vi "Roller Speeds.vi"(0 "Top In":dbl, 1 "Distance":dbl, 2 "Time Elapsed":bool, 3 "Selector":bool caption="Reset", 4 "Trigger":bool, 5 "Bottom In":dbl) -> (14 "Top Out":dbl, 19 "Bottom Out":dbl)   [LabVIEW 2012]
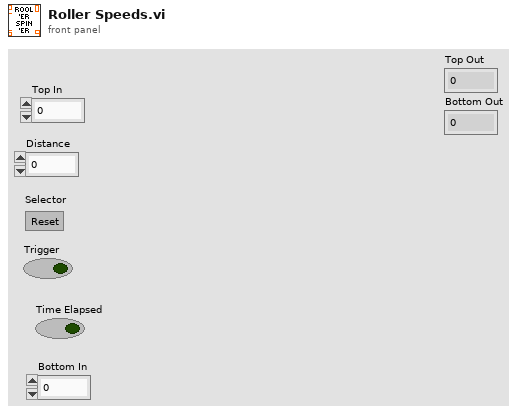
[diagram p1: front panel]
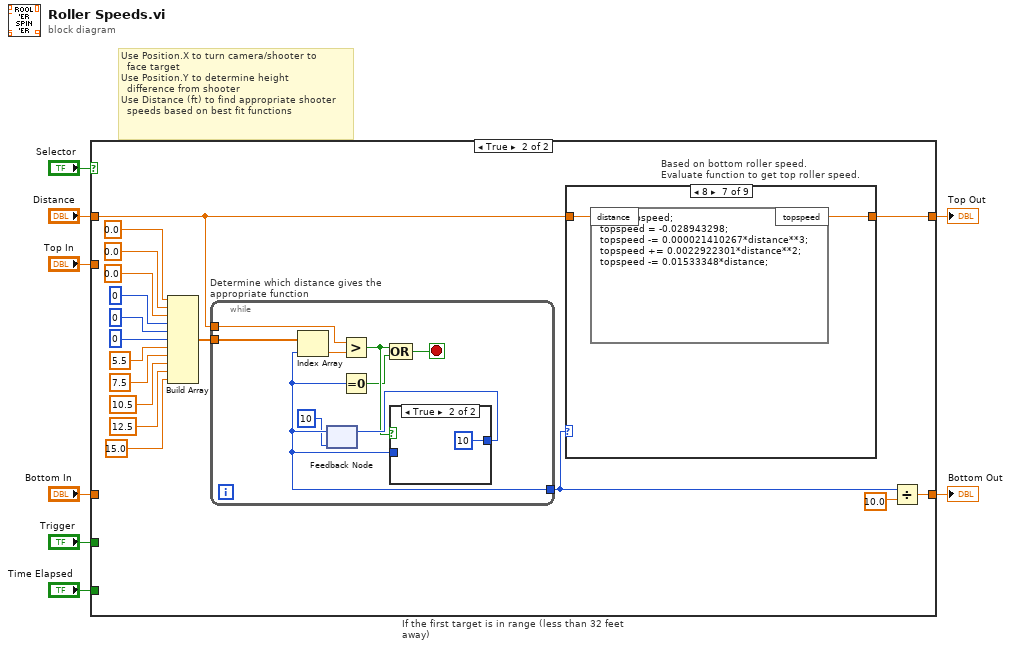
[diagram p0: block diagram]
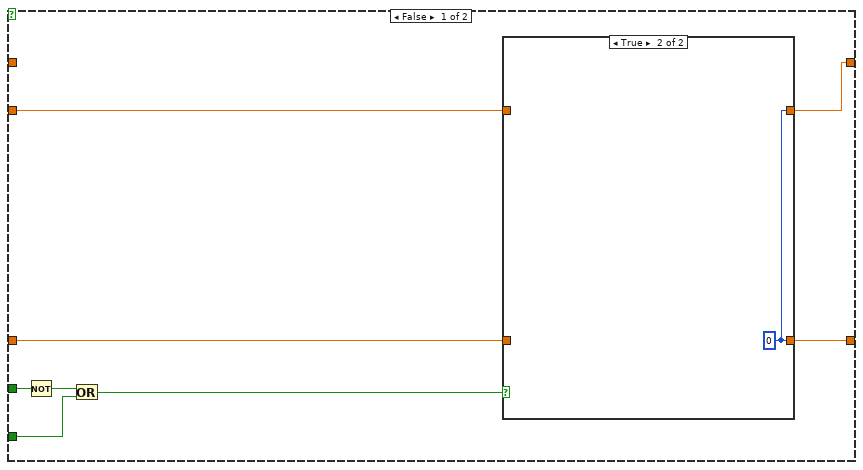
[diagram p2: hidden frame]
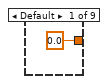
[diagram p4: hidden frame]
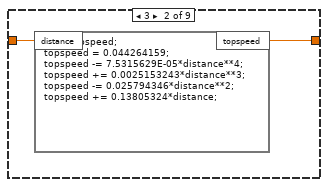
[diagram p5: hidden frame]
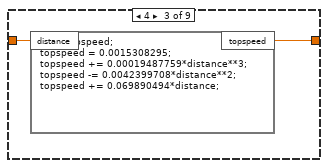
[diagram p6: hidden frame]
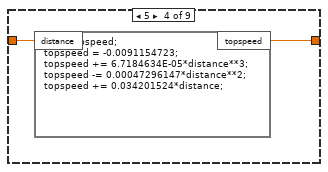
[diagram p7: hidden frame]
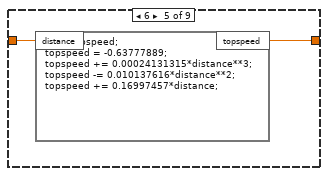
[diagram p8: hidden frame]
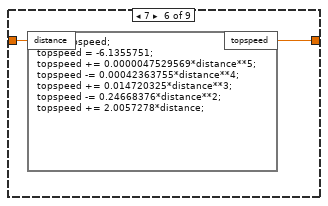
[diagram p9: hidden frame]
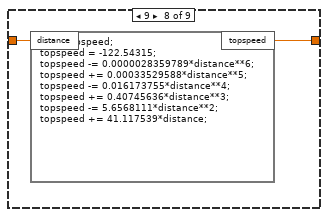
[diagram p10: hidden frame]
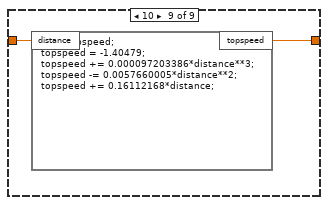
[diagram p11: hidden frame]
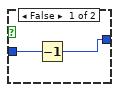
[diagram p12: hidden frame]
diagram:
  # "Use Position.X to turn camera/shooter to\n  face target\nUse Position.Y to determine height\n  difference from shooter\nUse Distance (ft) to find appropriate shooter\n  speeds based on best fit functions"
  n1 = case "If the first target is in range (less than 32 feet away)" shown="True" "Selector" {
    tunnel: [w16 w24] -> w6
    tunnel: [w15 w21] -> w7
    tunnel: "Top In" -> [w14 _]
    tunnel: "Bottom In" -> [w9 _]
    tunnel: "Time Elapsed" -> [w13 _]
    tunnel: "Trigger" -> [w10 _]
    tunnel: "Distance" -> [_ w20]
    frame False {
      n2 = Not(x=w10) -> (.not. x?=w11:bool)
      n3 = Or(x=w11, y=w13) -> (x .or. y?=w12:bool)
      n4 = case shown="True" w12 {
        tunnel: [w18 w19] -> w15
        tunnel: [w17 w19] -> w16
        tunnel: w14 -> [w18 _]
        tunnel: w9 -> [w17 _]
        frame False {
        }
        frame True {
          w19 = 0
        }
      }
    }
    frame True {
      n5 = Build Array(0.0, 0.0, 0.0, 0, 0, 0, 5.5, 7.5, 10.5, 12.5, 15.0 ("element")) -> (w25:dbl[])
      n6 = while "Determine which distance gives the appropriate function" {
        tunnel: w25 -> [w62]
        tunnel: [w57] -> w22
        tunnel: w20 -> [w55]
        stop <- w56 stop-if-true
        n7 = feedback #1(10) -> (w57:i32)
        n8 = Index Array(array=w62, index=w57) -> (element=w61:dbl)
        n9 = Greater?(x=w55, y=w61) -> (0:w59:bool)
        n10 = Equal To 0?(x=w57) -> (x = 0?=w58:bool)
        n11 = Compound Arithmetic op=OR(w59, w58) -> (w56:bool)
        n12 = case shown="True" w59 {
          tunnel: w57 -> [w64 _]
          tunnel: [w63 10] -> w60
          frame False {
            n13 = Decrement(x=w64) -> (x-1=w63:i32)
          }
          frame True {
          }
        }
        n14 = feedback-in #1(w60) -> ()
      }
      n15 = case "Based on bottom roller speed.\nEvaluate function to get top roller speed." shown="8" w22 {
        tunnel: [0.0 w39 w41 w43 w45 w47 w49 w51 w53] -> w21
        tunnel: w20 -> [_ w38 w40 w42 w44 w46 w48 w50 w52]
        frame Default {
        }
        frame 3 {
          n16 = formula code="float topspeed;\ntopspeed = 0.044264159;\ntopspeed -= 7.5315629E-05*distance**4;\ntopspeed += 0.0025153243*distance**3;\ntopspeed -= 0.025794346*distance**2;\ntopspeed += 0.13805324*distance;"("distance"=w38) -> ("topspeed"=w39:dbl)
        }
        frame 4 {
          n17 = formula code="float topspeed;\ntopspeed = 0.0015308295;\ntopspeed += 0.00019487759*distance**3;\ntopspeed -= 0.0042399708*distance**2;\ntopspeed += 0.069890494*distance;"("distance"=w40) -> ("topspeed"=w41:dbl)
        }
        frame 5 {
          n18 = formula code="float topspeed;\ntopspeed = -0.0091154723;\ntopspeed += 6.7184634E-05*distance**3;\ntopspeed -= 0.00047296147*distance**2;\ntopspeed += 0.034201524*distance;"("distance"=w42) -> ("topspeed"=w43:dbl)
        }
        frame 6 {
          n19 = formula code="float topspeed;\ntopspeed = -0.63777889;\ntopspeed += 0.00024131315*distance**3;\ntopspeed -= 0.010137616*distance**2;\ntopspeed += 0.16997457*distance;"("distance"=w44) -> ("topspeed"=w45:dbl)
        }
        frame 7 {
          n20 = formula code="float topspeed;\ntopspeed = -6.1355751;\ntopspeed += 0.0000047529569*distance**5;\ntopspeed -= 0.00042363755*distance**4;\ntopspeed += 0.014720325*distance**3;\ntopspeed -= 0.24668376*distance**2;\ntopspeed += 2.0057278*distance;"("distance"=w46) -> ("topspeed"=w47:dbl)
        }
        frame 8 {
          n21 = formula code="float topspeed;\ntopspeed = -0.028943298;\ntopspeed -= 0.000021410267*distance**3;\ntopspeed += 0.0022922301*distance**2;\ntopspeed -= 0.01533348*distance;"("distance"=w48) -> ("topspeed"=w49:dbl)
        }
        frame 9 {
          n22 = formula code="float topspeed;\ntopspeed = -122.54315;\ntopspeed -= 0.0000028359789*distance**6;\ntopspeed += 0.00033529588*distance**5;\ntopspeed -= 0.016173755*distance**4;\ntopspeed += 0.40745636*distance**3;\ntopspeed -= 5.6568111*distance**2;\ntopspeed += 41.117539*distance;"("distance"=w50) -> ("topspeed"=w51:dbl)
        }
        frame 10 {
          n23 = formula code="float topspeed;\ntopspeed = -1.40479;\ntopspeed += 0.000097203386*distance**3;\ntopspeed -= 0.0057660005*distance**2;\ntopspeed += 0.16112168*distance;"("distance"=w52) -> ("topspeed"=w53:dbl)
        }
      }
      n24 = Divide(x=w22, y=10.0) -> (x/y=w24:dbl)
    }
  }
  "Top Out" <- w7
  "Bottom Out" <- w6
